vi "LPA400_get_rdg.vi"(4 "Channel Name":string, 7 "Address":T1={"Main"=99, "Ch."=1, "Sub"=3, "Port Name"="Belkin USB Serial Adapter"}) -> (0 "Output":dbl=nan format="%.2f", 3 "Status note":string)   [LabVIEW 2010]
uses:
  ADAM Client/Sub VIs/ADAM Controls/Address.ctl
  ADAM Client/Sub VIs/ADAM Controls/Remember_value_mode.ctl
panel:
  out "Read":string
  # "Main=0 for direct connection, otherwise Main=address of 4521.\nSub indicates number of channels attached- required for serial termination\nChannel is required channel number."
  # "Test String: #X01+11FI!#X02+22FL!#X03+33FO!"
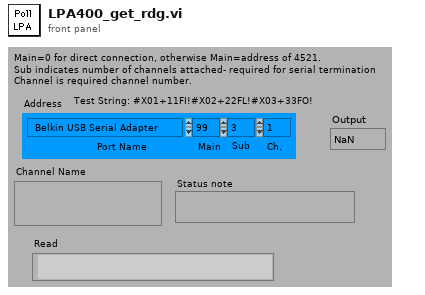
[diagram p1: front panel]
types:
  T1 = typedef "Address.ctl" = cluster{"Main":i32, "Ch.":i32, "Sub":i32, "Port Name":string}
  T2 = typedef "Remember_value_mode.ctl" = enum16{"Read only", "Read and Write"}
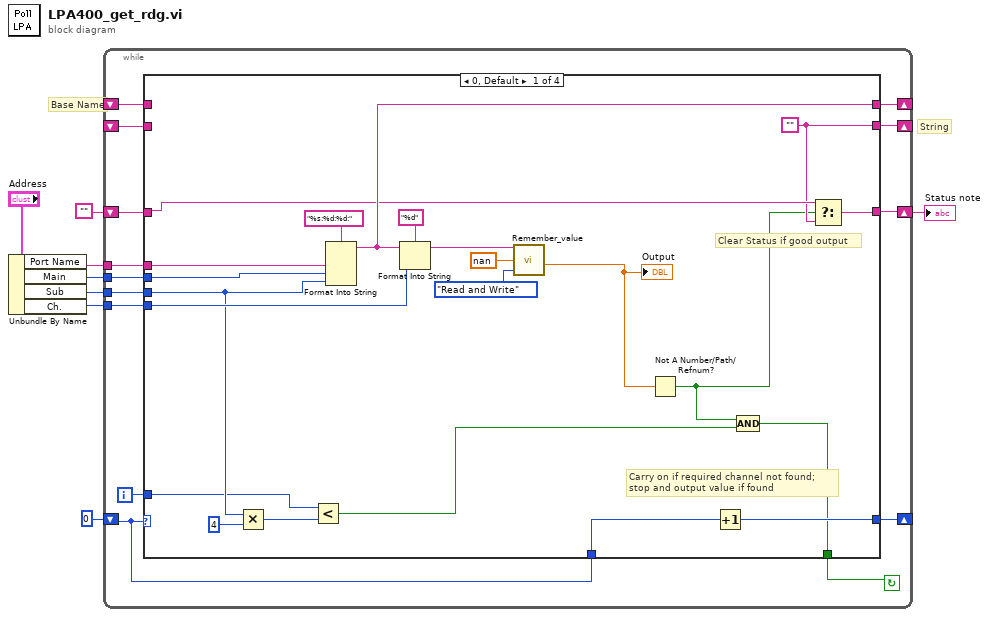
[diagram p0: block diagram]
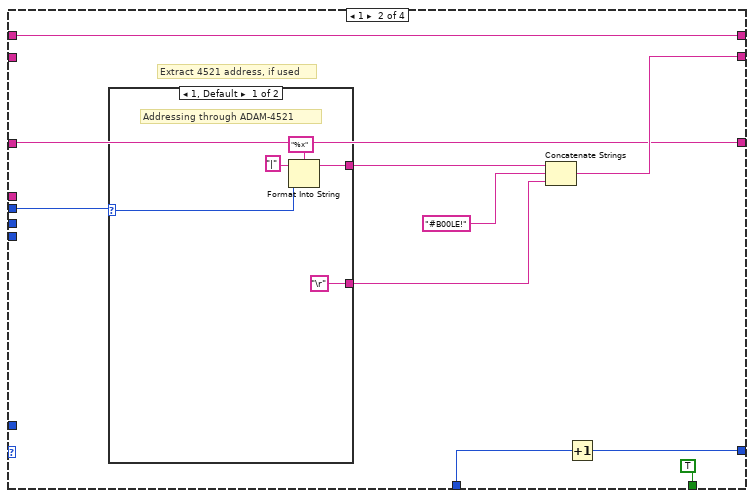
[diagram p2: hidden frame]
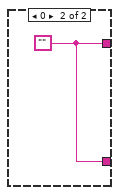
[diagram p3: hidden frame]
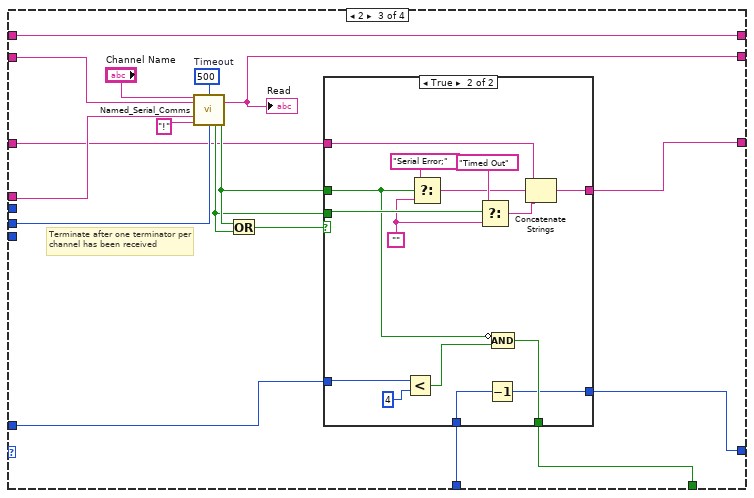
[diagram p4: hidden frame]
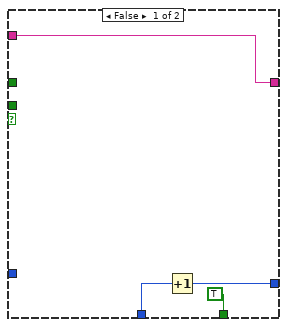
[diagram p5: hidden frame]
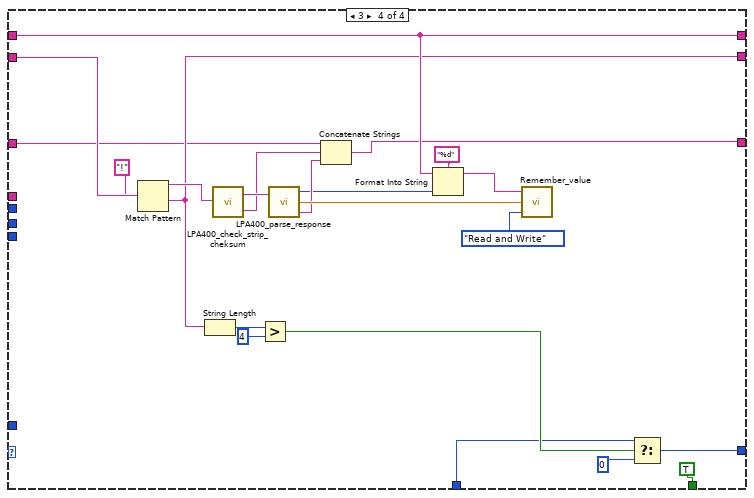
[diagram p6: hidden frame]
diagram:
  # "Base Name"
  # "String"
  n1 = Unbundle By Name("Address") -> ("Port Name"=w5:string, "Main"=w6:i32, "Sub"=w4:i32, "Ch."=w3:i32)
  n2 = while {
    tunnel: w3 -> [w11]
    tunnel: w4 -> [w12]
    tunnel: w5 -> [w13]
    tunnel: w6 -> [w14]
    shift-left: "" -> [w9]
    shift-right: [w10] -> w1
    shift-left: _ -> [w17]
    shift-right: [w18] -> _
    shift-left: _ -> [w16]
    shift-right: [w21] -> _
    shift-left: 0 -> [w15]
    shift-right: [w22] -> _
    i -> [w19]
    stop <- w20 continue-if-true
    n3 = case shown="0, Default" w15 {
      tunnel: w15 -> [w40 w49 w74 w101]
      tunnel: [w41 w47 w73 w99] -> w22
      tunnel: [w35 w54 w69 w111] -> w21
      tunnel: [w23 TRUE w71 TRUE] -> w20
      tunnel: w19 -> [w26 _ w72 _]
      tunnel: [w31 w53 w70 w110] -> w18
      tunnel: w17 -> [_ _ w65 w118]
      tunnel: w16 -> [_ w54 w69 w111]
      tunnel: w14 -> [w38 w46 _ _]
      tunnel: w13 -> [w39 _ w64 _]
      tunnel: w12 -> [w27 _ w63 _]
      tunnel: w11 -> [w37 _ _ _]
      tunnel: [w33 w45 w62 w103] -> w10
      tunnel: w9 -> [w32 w45 w61 w104]
      frame 0, Default {
        w31 = ""
        # "Clear Status if good output"
        # "Carry on if required channel not found;\nstop and output value if found"
        n4 = Multiply(x=w27, y=4) -> (x*y=w28:i32)
        n5 = Less?(x=w26, y=w28) -> (x < y?=w25:bool)
        n6 = Format Into String(format string="%s:%d:%d:" ("Format String"), w39, w38, w27) -> (resulting string=w35:string)  [unwired: 2 in, 1 out]
        n7 = Format Into String(format string="%d" ("Format String"), initial string=w35, w37) -> (resulting string=w34:string)  [unwired: 1 in, 1 out]
        n8 = call "Remember_value.vi"("Mode"=Remember_value_mode."Read and Write", "Input Value"=nan, "Ch name"=w34) -> ("Output Value"=w30:dbl)
        "Output" <- w30
        n9 = Not A Number/Path/Refnum?(number/path/refnum=w30) -> (NaN/Path/Refnum?=w24:bool)
        n10 = Increment(x=w40) -> (x+1=w41:i32)
        n11 = Compound Arithmetic op=AND(w24, w25) -> (w23:bool)
        n12 = Select(t=w32, s=w24, f=w31) -> (s? t:f=w33:string)
      }
      frame 1 {
        # "Extract 4521 address, if used"
        n13 = case shown="1, Default" w46 {
          selector: w46 -> [w55 _]
          tunnel: [w56 w60] -> w51
          tunnel: ["\r" w60] -> w52
          frame 1, Default {
            # "Addressing through ADAM-4521"
            n14 = Format Into String(format string="%x" ("Format String"), initial string="|" ("Substring"), w55) -> (resulting string=w56:string)  [unwired: 1 in, 1 out]
          }
          frame 0 {
            w60 = ""
          }
        }
        n15 = Concatenate Strings(w51, "#B00LE!", w52) -> (w53:string)
        n16 = Increment(x=w49) -> (x+1=w47:i32)
      }
      frame 2 {
        w77 = u32 500  # Timeout
        # "Terminate after one terminator per channel has been received"
        n17 = call "Named_Serial_Comms.vi"("Channel Name"="Channel Name", "Write String"=w65, "Timeout/ms"=w77, "Port Name"=w64, "Term Grep"="!", "Terminate Count"=w63) -> ("Read"=w70:string, "Timed out"=w67:bool, "Serial Error"=w68:bool)  [unwired: 3 in, 4 out]
        "Read" <- w70
        n18 = Or(x=w68, y=w67) -> (x .or. y?=w75:bool)
        n19 = case shown="True" w75 {
          tunnel: w68 -> [_ w87]
          tunnel: w67 -> [_ w96]
          tunnel: w74 -> [w80 w85]
          tunnel: [w79 w82] -> w73
          tunnel: w72 -> [_ w90]
          tunnel: [TRUE w86] -> w71
          tunnel: [w78 w84] -> w62
          tunnel: w61 -> [w78 w83]
          frame False {
            n20 = Increment(x=w80) -> (x+1=w79:i32)
          }
          frame True {
            w91 = ""
            n21 = Less?(x=w90, y=4) -> (x < y?=w88:bool)
            n22 = Select(t="Serial Error;", s=w87, f=w91) -> (s? t:f=w93:string)
            n23 = Select(t="Timed Out", s=w96, f=w91) -> (s? t:f=w92:string)
            n24 = Decrement(x=w85) -> (x-1=w82:i32)
            n25 = Compound Arithmetic op=AND(invert w87, w88) -> (w86:bool)
            n26 = Concatenate Strings(w83, w93, w92) -> (w84:string)
          }
        }
      }
      frame 3 {
        n27 = Match Pattern(string=w118, regular expression="!" ("Format String")) -> (before substring=w116:string, after substring=w110:string)  [unwired: 3 out]
        n28 = String Length(string=w110) -> (length=w109:i32)
        n29 = call "LPA400_check_strip_cheksum.vi"("LPA400 individual scale string"=w116) -> ("Cleaned good string"=w115:string, "Error Notes"=w113:string)
        n30 = Greater?(x=w109, y=4) -> (0:w102:bool)
        n31 = call "LPA400_parse_response.vi"("Stripped scale response"=w115) -> ("Address"=w98:i32, "Weight"=w114:dbl, "Error notes"=w112:string)
        n32 = Concatenate Strings(w104, w113, w112) -> (w103:string)
        n33 = Format Into String(format string="%d" ("Format String"), initial string=w111, w98) -> (resulting string=w105:string)  [unwired: 1 in, 1 out]
        n34 = call "Remember_value.vi"("Mode"=Remember_value_mode."Read and Write", "Input Value"=w114, "Ch name"=w105) -> ()  [unwired: 1 out]
        n35 = Select(t=w101, s=w102, f=0) -> (s? t:f=w99:i32)
      }
    }
  }
  "Status note" <- w1
